vi "Result To String2.vi"(10 "CmdName":string, 11 "Result":refnum<vi>) -> (3 "SendCmd":string)   [LabVIEW 2019]
uses:
  Function/VisionSet/System/iVision/Controls/Parameter.ctl
  2f1d9a6e-04d9-4eca-a5af-4b65213a62f9.vi
  <vilib>/JDP Science/JSONtext/JSON text to Variant.vi
  <vilib>/vision/NI_Vision_Development_Module.lvlib
panel:
  out "OK":bool
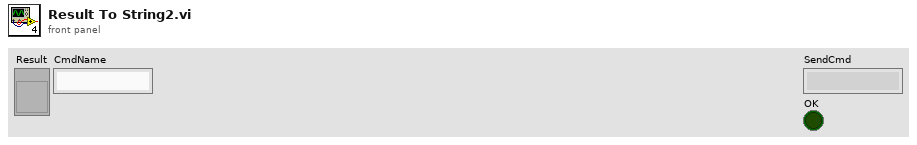
[diagram p1: front panel]
types:
  T1 = cluster{"ROI":string, "Numbers":i32, "Data":string[][]}[]
  T2 = cluster{"ROI":string, "Numbers":i32, "Data":string[][]}
  T3 = typedef "Parameter.ctl" = enum16{"Initialize", "Write", "Read", "WriteAll", "Save", "Load"}
  T4 = enum16{"Initial", "Write", "Read", "Save", "Load", "WrteAll"}
  T5 = typedef "ParameterData.ctl" = cluster{"Rotate Angle":dbl, "Rotate?":bool, "Calibration File Path":string, "Cal?":bool}
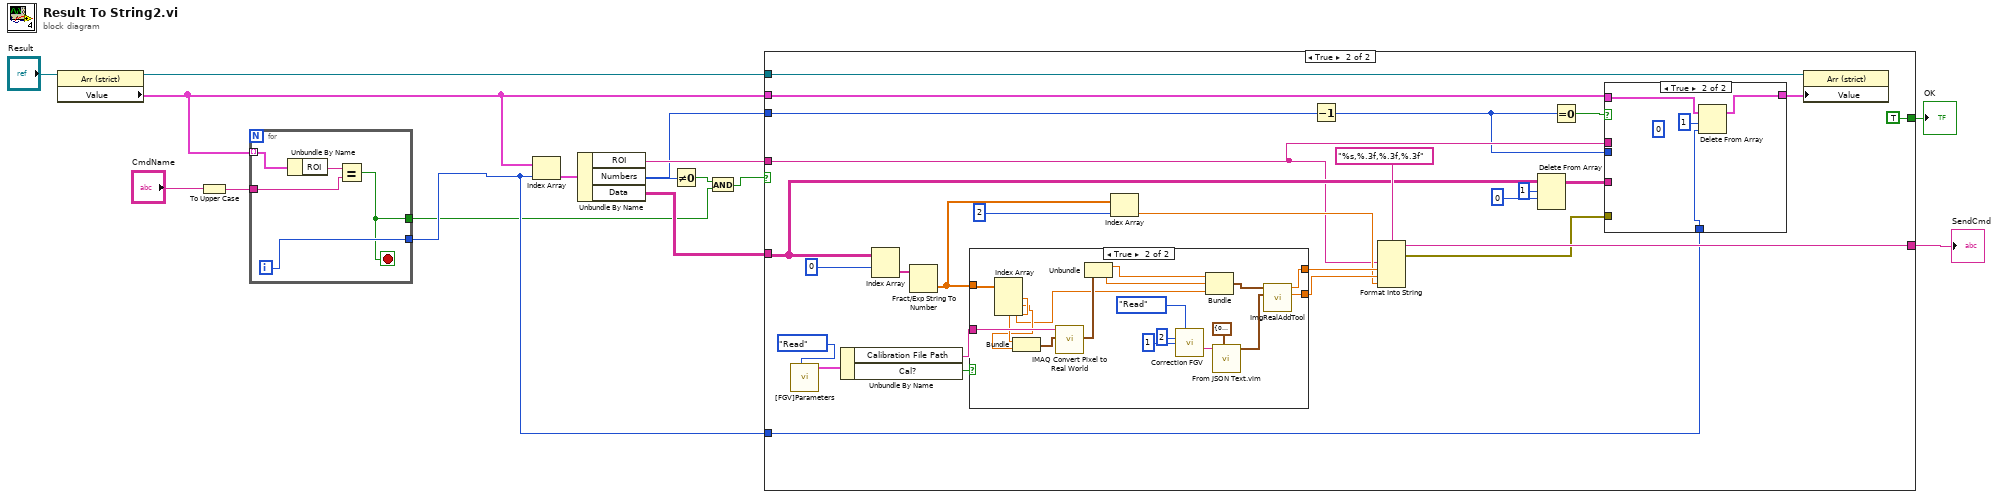
[diagram p0: block diagram]
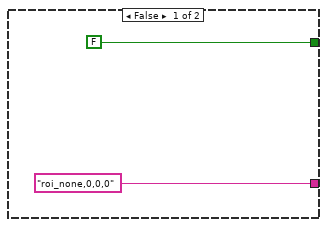
[diagram p2: hidden frame]
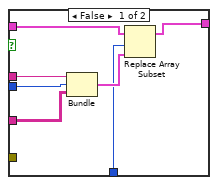
[diagram p3: hidden frame]
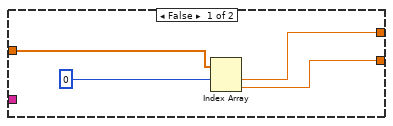
[diagram p4: hidden frame]
diagram:
  n1 = property class="Arr (strict)"(reference="Result") -> (reference out=w11:refnum<vi>, "Value"=w7:T1)  [unwired: 1 in, 1 out]
  n2 = To Upper Case(1:"CmdName") -> (0:w4:string)
  n3 = for {
    tunnel: w7 -> [w20] mode=indexing
    tunnel: [w18] -> w6
    tunnel: w4 -> [w17]
    tunnel: [w16] -> w1
    i -> [w18]
    stop <- w16 stop-if-true
    n4 = Unbundle By Name(w20) -> ("ROI"=w19:string)
    n5 = Equal?(x=w19, y=w17) -> (x = y?=w16:bool)
  }
  n6 = Index Array(array=w7, index=w6) -> (element=w15:T2)
  n7 = Unbundle By Name(w15) -> ("ROI"=w13:string, "Numbers"=w10:i32, "Data"=w14:string[][])
  n8 = Not Equal To 0?(x=w10) -> (x != 0?=w3:bool)
  n9 = And(x=w3, y=w1) -> (x .and. y?=w2:bool)
  n10 = case shown="True" w2 {
    tunnel: w14 -> [_ w36]
    tunnel: w13 -> [_ w28]
    tunnel: ["roi_none,0,0,0" w38] -> w9
    tunnel: w11 -> [_ w33]
    tunnel: w10 -> [_ w37]
    tunnel: w7 -> [_ w31]
    tunnel: [FALSE TRUE] -> w8
    tunnel: w6 -> [_ w23]
    frame False {
    }
    frame True {
      n11 = call "[FGV]Parameters.vi"("Parameter"=Parameter."Read") -> ("ParameterData Out"=w41:T5)  [unwired: 9 in, 1 out]
      n12 = Unbundle By Name(w41) -> ("Calibration File Path"=w24:string, "Cal?"=w39:bool)
      n13 = Index Array(array=w36, index (row)=0) -> (element=w48:string[])  [unwired: 1 in]
      n14 = Fract/Exp String To Number(string=w48) -> (number=w47:dbl[])  [unwired: 3 in, 1 out]
      n15 = case shown="True" w39 {
        tunnel: w47 -> [w63 w74]
        tunnel: [w62 w76] -> w44
        tunnel: [w61 w75] -> w43
        tunnel: w24 -> [_ w73]
        frame False {
          n16 = Index Array(array=w63, index #1=0 ("index")) -> (element #1=w62:dbl, element #2=w61:dbl)  [unwired: 1 in]
        }
        frame True {
          n17 = Index Array(array=w74) -> (element #1=w72:dbl, element #2=w71:dbl, element #3=w66:dbl)  [unwired: 3 in]
          n18 = Bundle(w72, w71) -> (w70:cluster{dbl, dbl})  [unwired: 1 in]
          n19 = call "IMAQ Convert Pixel to Real World"("Pixel Coordinates"=w70, "Calibrated Image"=w73) -> ("Real World Coordinates"=w69:cluster{"X":sgl, "Y":sgl})  [unwired: 4 in, 5 out]
          n20 = Unbundle(w69) -> ("X"=w68:sgl, "Y"=w67:sgl)
          n21 = call "Correction FGV.vi"("Action"=T4."Read", "X"=2, "Y"=1) -> ("DataOut"=w82:string)  [unwired: 10 in, 2 out]
          n22 = Bundle("X"=w68, "Y"=w67, w66) -> (w65:cluster{"X":sgl, "Y":sgl, dbl})  [unwired: 1 in]
          n23 = call "From JSON Text.vim"("Data Type and Default Value"=cluster{"X":dbl, "Y":dbl, "Angle":dbl} {"X"=0.0, "Y"=0.0, "Angle"=0.0} ("ToolData"), "JSON"=w82) -> ("Data out"=w77:cluster{"X":dbl, "Y":dbl, "Angle":dbl})  [unwired: 8 in, 1 out]
          n24 = call "ImgRealAddTool.vi"("ToolData"=w77, "ImgRealData"=w65) -> ("YFinal"=w75:dbl, "XFinal"=w76:dbl)  [unwired: 8 in]
        }
      }
      n25 = Index Array(array=w47, index=2) -> (element=w42:dbl)
      n26 = Decrement(x=w37) -> (x-1=w27:i32)
      n27 = Format Into String(format string="%s,%.3f,%.3f,%.3f", w28, w44, w43, w42) -> (resulting string=w38:string, error out=w29:errorcluster)  [unwired: 2 in]
      n28 = Delete From Array(array=w36, length=1, index (row)=0) -> (array with subset deleted=w26:string[][])  [unwired: 1 in, 1 out]
      n29 = Equal To 0?(x=w27) -> (x = 0?=w32:bool)
      n30 = case shown="True" w32 {
        tunnel: w31 -> [w55 w59]
        tunnel: [w56 w58] -> w30
        tunnel: w29 -> [_ _]
        tunnel: w28 -> [w54 _]
        tunnel: w27 -> [w53 _]
        tunnel: w26 -> [w52 _]
        tunnel: w23 -> [w50 w57]
        frame False {
          n31 = Bundle("ROI"=w54, w53, "Data"=w52) -> (w51:cluster{"ROI":string, i32, "Data":string[][]})  [unwired: 1 in]
          n32 = Replace Array Subset(array=w55, new element=w51, index=w50) -> (w56:T1)
        }
        frame True {
          (unwired) 0 ("index (row)")
          n33 = Delete From Array(array=w59, length=1, index=w57) -> (array with subset deleted=w58:T1)  [unwired: 1 out]
        }
      }
      n34 = property class="Arr (strict)"(reference=w33, "Value"=w30) -> ()  [unwired: 1 in, 2 out]
    }
  }
  "SendCmd" <- w9
  "OK" <- w8
